vi "CalcDiff.vi"(8 "error in (no error)":errorcluster, 11 "XYZ Point coordinates (pixels)":dbl[][](array[numeric])) -> (0 "error out":errorcluster, 3 "XYZ Point coordinates (pixels) difference":dbl[][](array[numeric]))   [LabVIEW 2010]
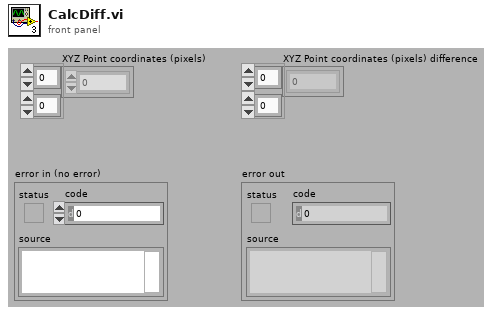
[diagram p1: front panel]
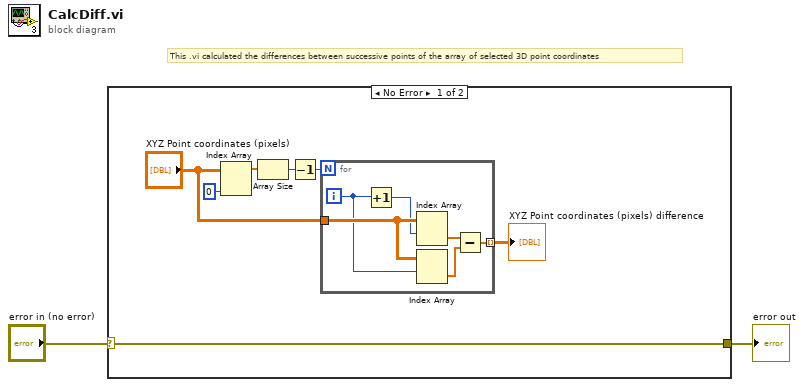
[diagram p0: block diagram]
diagram:
  # "This .vi calculated the differences between successive points of the array of selected 3D point coordinates"
  n1 = case shown="No Error" "error in (no error)" {
    selector: "error in (no error)" -> [w3 w16]
    tunnel: [w3 w16] -> w1
    frame No Error {
      n2 = Index Array(array="XYZ Point coordinates (pixels)", index (col)=0 ("disabled index (col)")) -> (element=w8:dbl[])  [unwired: 1 in]
      n3 = Array Size(array=w8) -> (size(s)=w6:i32)
      n4 = Decrement(x=w6) -> (x-1=w7:i32)
      n5 = for {
        N: w7 -> [_]
        tunnel: "XYZ Point coordinates (pixels)" -> [w15]
        tunnel: [w10] -> w4 mode=indexing
        i -> [w13]
        n6 = Increment(x=w13) -> (x+1=w14:i32)
        n7 = Index Array(array=w15, index (row)=w14) -> (element=w12:dbl[])  [unwired: 1 in]
        n8 = Index Array(array=w15, index (row)=w13) -> (element=w11:dbl[])  [unwired: 1 in]
        n9 = Subtract(x=w12, y=w11) -> (x-y=w10:dbl[])
      }
      "XYZ Point coordinates (pixels) difference" <- w4
    }
    frame Error {
    }
  }
  "error out" <- w1
